vi "Parse Table Column as JSON Array.vi"(7 "SpreadsheetDocument in":refnum<k24>, 8 "error in":errorcluster, 9 "Cells":variant[](array[variant]), 10 "Named Range":string, 11 "<JSON>":string="{}") -> (0 "error out":errorcluster, 3 "<JSON> out":string)   [LabVIEW 2020, in "Config from EXCEL.lvclass"]
uses:
  Config from EXCEL.lvclass
  D:/git/Open-Xml-LabVIEW/Source/DocumentFormat.OpenXml.dll
  Open-Xml-LabVIEW/Source/DocumentFormat.OpenXml.dll
  <vilib>/JDP Science/JSONtext/LVClass Serializer/JSONtext LVClass Serializer.lvclass
  Config from EXCEL.lvclass/Config from EXCEL.ctl
  <vilib>/JDP Science/JSONtext/JSONtext.lvlib
  3d530874-43db-4d28-b45c-a44206ee6d76.vi
  Open-Xml-LabVIEW/Source/Open Xml.lvlib
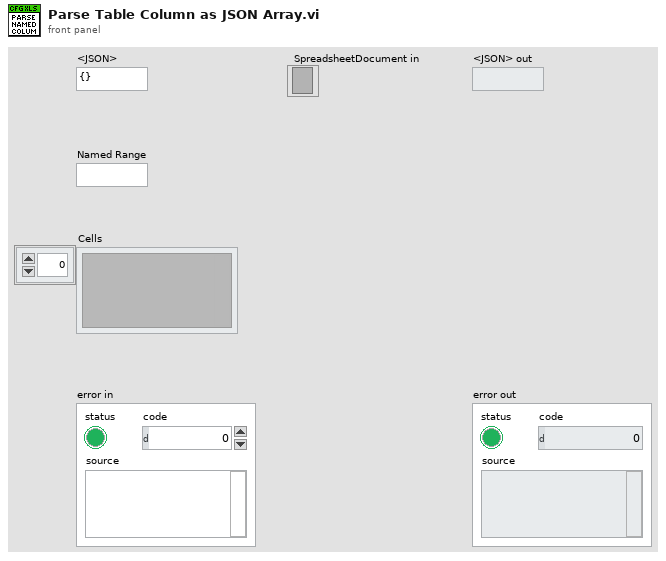
[diagram p1: front panel]
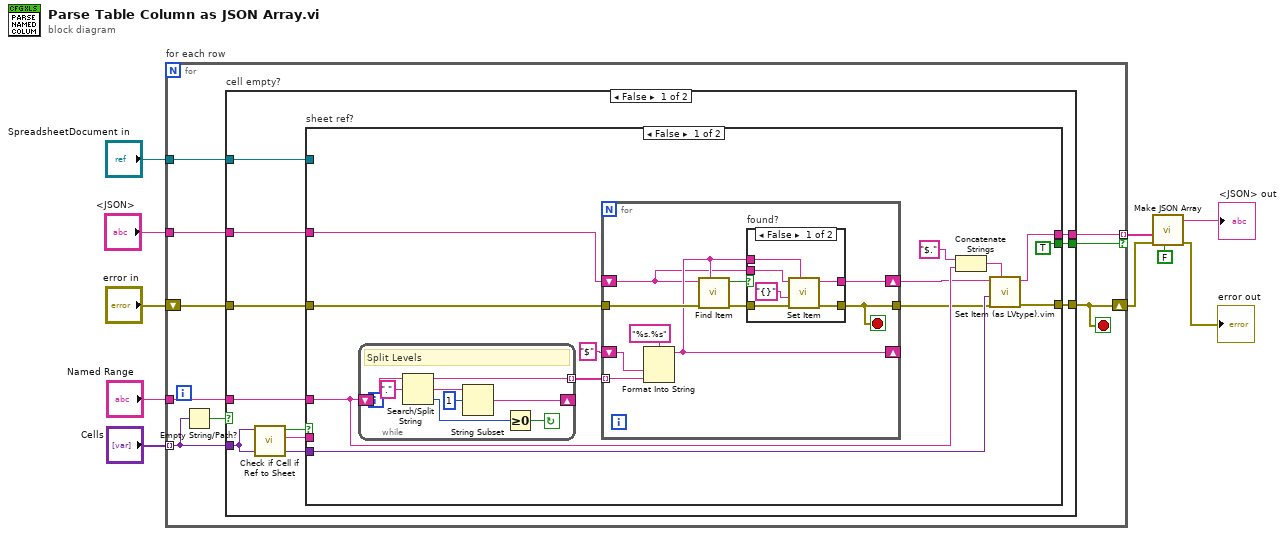
[diagram p0: block diagram]
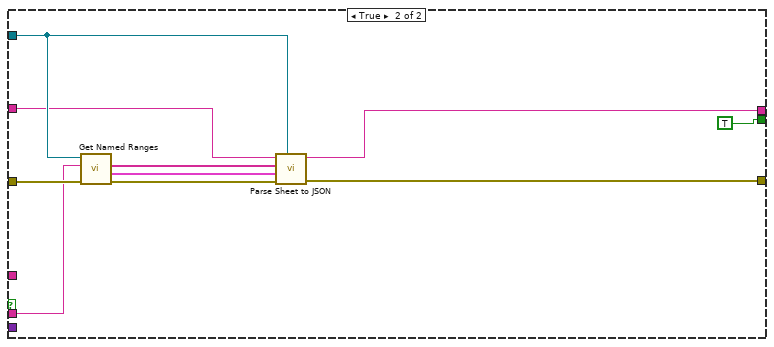
[diagram p3: hidden frame]
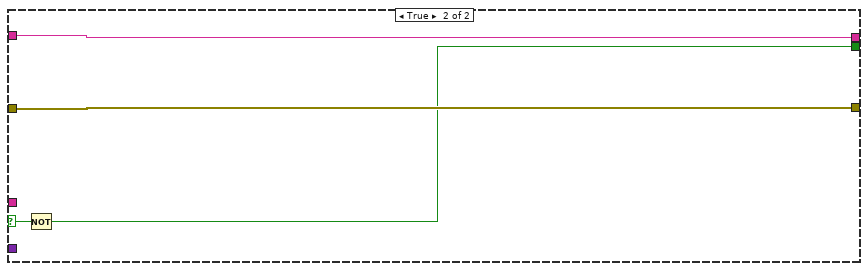
[diagram p4: hidden frame]
diagram:
  n1 = for "for each row" {
    tunnel: "Cells" -> [w12] mode=indexing
    tunnel: "SpreadsheetDocument in" -> [w18]
    shift-right: [w14] -> w2
    shift-left: "error in" -> [w19]
    tunnel: "Named Range" -> [w16]
    tunnel: "<JSON>" -> [w17]
    tunnel: [w15] -> w5 mode=indexing if=w13
    stop <- w14 stop-if-true
    n2 = Empty String/Path?(string/path=w12) -> (empty?=w11:bool)
    n3 = case "cell empty?" shown="False" w11 {
      selector: w11 -> [_ w80]
      tunnel: w19 -> [w29 w82]
      tunnel: w18 -> [w28 _]
      tunnel: w12 -> [w25 _]
      tunnel: w17 -> [w24 w81]
      tunnel: w16 -> [w23 _]
      tunnel: [w22 w82] -> w14
      tunnel: [w21 w81] -> w15
      tunnel: [w20 w79] -> w13
      frame False {
        n4 = call "Check if Cell if Ref to Sheet.vi"("Value"=w25) -> ("Sheet Name"=w27:string, "Sheet Ref"=w26:bool)  [unwired: 9 in]
        n5 = case "sheet ref?" shown="False" w26 {
          tunnel: w29 -> [w34 w78]
          tunnel: w28 -> [_ w71]
          tunnel: w27 -> [_ w77]
          tunnel: [w38 w75] -> w22
          tunnel: w25 -> [w40 _]
          tunnel: w24 -> [w31 w70]
          tunnel: w23 -> [w37 _]
          tunnel: [w39 w74] -> w21
          tunnel: [TRUE TRUE] -> w20
          frame False {
            n6 = while {
              shift-right: [w63] -> _
              shift-left: w37 -> [w62]
              tunnel: [w61] -> w36 mode=indexing
              stop <- w64 continue-if-true
              # "Split Levels"
              n7 = Search/Split String(string=w62, search string/char (-)=".") -> (substring before match=w61:string, match + rest of string=w65:string, offset of match=w67:i32)  [unwired: 1 in]
              n8 = String Subset(string=w65, offset (0)=1) -> (substring=w63:string)  [unwired: 1 in]
              n9 = Greater Or Equal To 0?(x=w67) -> (x >= 0?=w64:bool)
            }
            n10 = for {
              tunnel: w36 -> [w50] mode=indexing
              shift-right: [w45] -> _
              shift-left: "$" -> [w51]
              tunnel: w34 -> [w48]
              tunnel: [w47] -> w33
              shift-right: [w44] -> w32
              shift-left: w31 -> [w43]
              stop <- w47 stop-if-true
              n11 = Format Into String(format string="%s.%s", w51, w50) -> (resulting string=w45:string)  [unwired: 2 in, 1 out]
              n12 = call <vilib>:"Find Item.vi"("$Path or Item Name"=w45, "error in (no error)"=w48, "JSON"=w43) -> ("error out"=w49:errorcluster, "Found"=w46:bool)  [unwired: 5 in, 2 out]
              n13 = case "found?" shown="False" w46 {
                tunnel: [w57 w59] -> w44
                tunnel: [w56 w60] -> w47
                tunnel: w49 -> [w55 w60]
                tunnel: w45 -> [w54 _]
                tunnel: w43 -> [w53 w59]
                frame False {
                  n14 = call <vilib>:"Set Item.vi"("$Path or Item Name"=w54, "error in (no error)"=w55, "JSON to Insert"="{}", "JSON"=w53) -> ("error out"=w56:errorcluster, "<JSON>"=w57:string)  [unwired: 4 in, 1 out]
                }
                frame True {
                }
              }
            }
            n15 = Concatenate Strings("$." ("string"), w37) -> (w41:string)
            n16 = call "Set Item (as LVtype).vim"("$Path or Item Name"=w41, "error in (no error)"=w33, "Anything"=w40, "JSON"=w32) -> ("error out"=w38:errorcluster, "<JSON>"=w39:string)  [unwired: 4 in, 1 out]
          }
          frame True {
            n17 = call "Get Named Ranges.vi"("error in"=w78, "Sheet Name"=w77, "SpreadsheetDoc in"=w71) -> ("error out"=w76:errorcluster, "Cells"=w73:cluster{"Cells":variant[][]}[], "Range Names"=w72:string[])  [unwired: 5 in, 1 out]
            n18 = call "Parse Sheet to JSON.vi"("SpreadsheetDocument in"=w71, "error in"=w76, "Cells"=w73, "Named Ranges"=w72, "<JSON> in"=w70) -> ("error out"=w75:errorcluster, "<JSON> out"=w74:string)  [unwired: 5 in]
          }
        }
      }
      frame True {
        n19 = Not(x=w80) -> (.not. x?=w79:bool)
      }
    }
  }
  n20 = call <vilib>:"Make JSON Array.vi"("Pretty Print?"=FALSE, "error in (no error)"=w2, "JSON Elements"=w5) -> ("error out"=→"error out":errorcluster, "<JSON>"=→"<JSON> out":string)  [unwired: 7 in]
